vi "NT_LL_Read String.vi"(8 "error in (no error)":errorcluster, 10 "default value":string, 11 "subscribeHandle":u32) -> (0 "error out":errorcluster, 2 "time":i64, 3 "value":string)   [LabVIEW 2025]
uses:
  FRC_NetworkTablesLV.dll
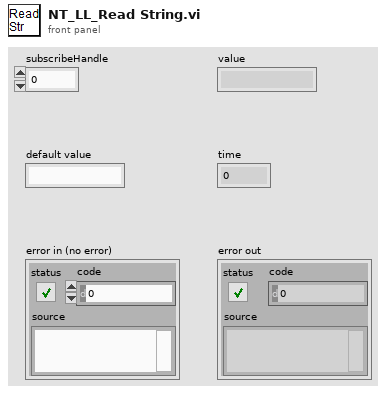
[diagram p1: front panel]
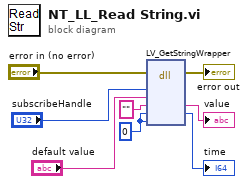
[diagram p0: block diagram]
diagram:
  w8 = i64 0 ("serverTime")
  n1 = dll-call lib="FRC_NetworkTablesLV.*" fn="LV_GetStringWrapper"(error in="error in (no error)", "subscribeHandle"="subscribeHandle", "default"="default value", "value"="", "time"=w8, "serverTime"=w8) -> (error out=→"error out":errorcluster, "value"=→"value":string, "time"=→"time":i64)  [unwired: 6 in, 1 out]
